vi "Rotation3D_Create_RotMatrix.vi"(11 "RotationMatrix":T1) -> (0 "Error":bool, 3 "Rotation3d":T2={"Q_quaternion"={"R"=1.0, "V"=[0.0, 0.0, 0.0]}})   [LabVIEW 2019, in "Trajectory_Library.lvlib"]
doc: "Constructs a Rotation3d from a rotation matrix.\n\nInputs::\n -- rotationMatrix -- The rotation matrix\n\nReturns:\n -- Rotation3d -- The created Rotation3d data cluster\n -- Error -- TRUE indicates an error occured."
uses:
  Trajectory_Library.lvlib
  TypeDef/ROTATION3D.ctl
  TypeDef/QUATERNION.ctl
  <vilib>/Analysis/Matrix/Datatypes/RealMatrix.ctl
  <vilib>/Analysis/baseanly.llb/Real A x B.vi
  <vilib>/Analysis/baseanly.llb/Real Determinant.vi
  Quaternion_Normalize.vi
  Quaternion_New_Default.vi
  <vilib>/Analysis/7linalg.llb/Create Special Matrix.vi
  <vilib>/Analysis/7linalg.llb/Create Special Real Matrix.vi
  <vilib>/Analysis/NI_AALBase.lvlib
  <vilib>/Analysis/Matrix/NI_Matrix.lvlib
  <vilib>/Analysis/Matrix/Numeric/Subtract/Subtract - RM,RM.vi
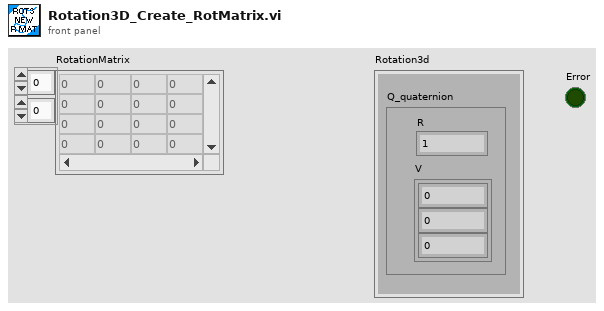
[diagram p1: front panel]
types:
  T1 = typedef "NI_Matrix.lvlib/RealMatrix.ctl" = dbl[][]
  T2 = typedef "Trajectory_Library.lvlib/ROTATION3D.ctl" = cluster{"Q_quaternion":T3}
  T3 = typedef "Trajectory_Library.lvlib/QUATERNION.ctl" = cluster{"R":dbl, "V":dbl[]}
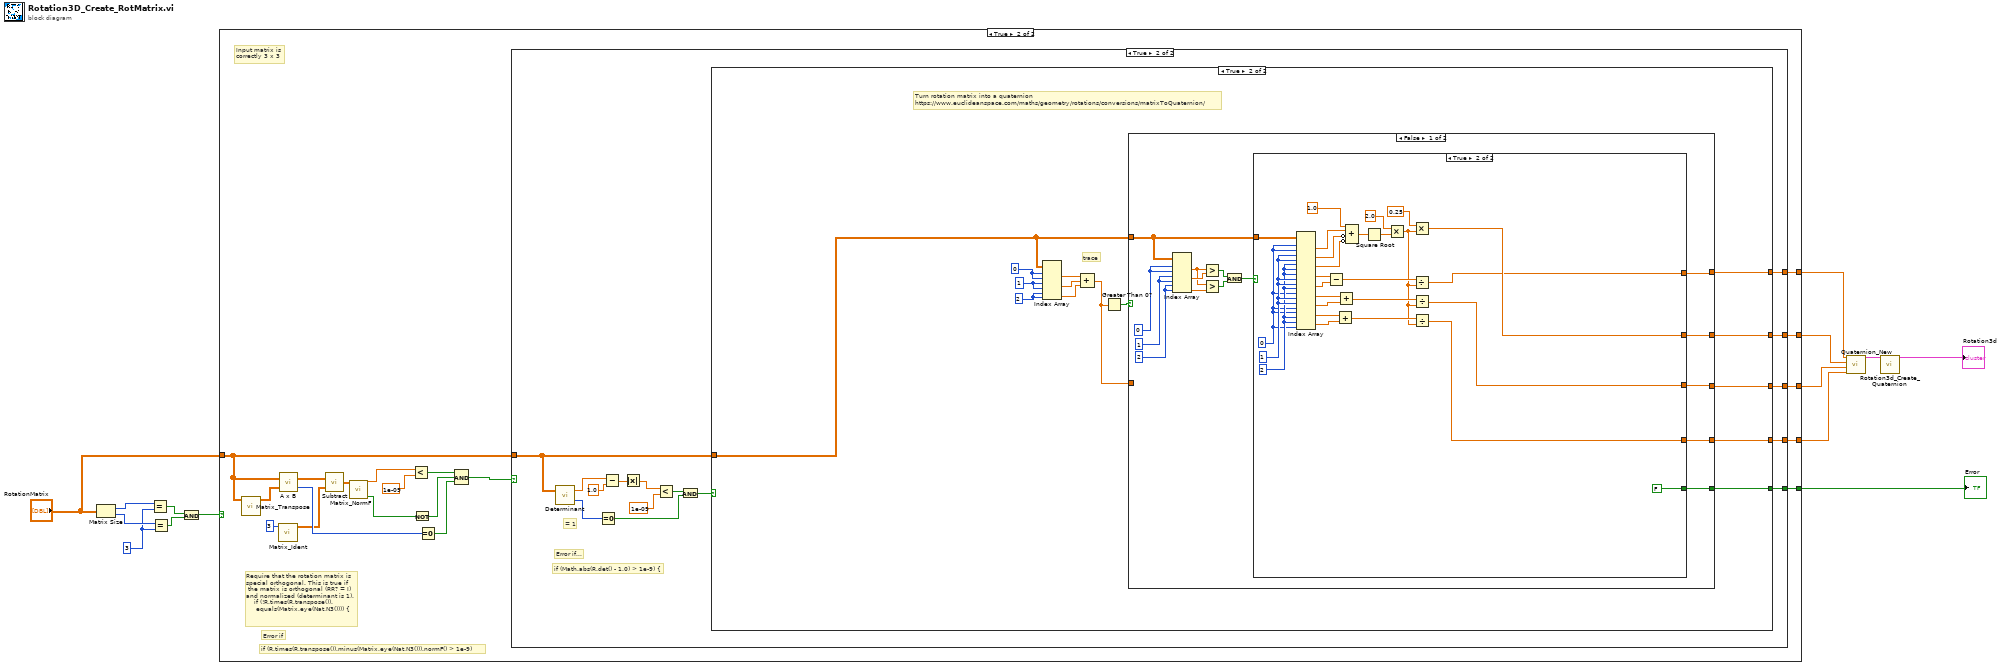
[diagram p0: block diagram]
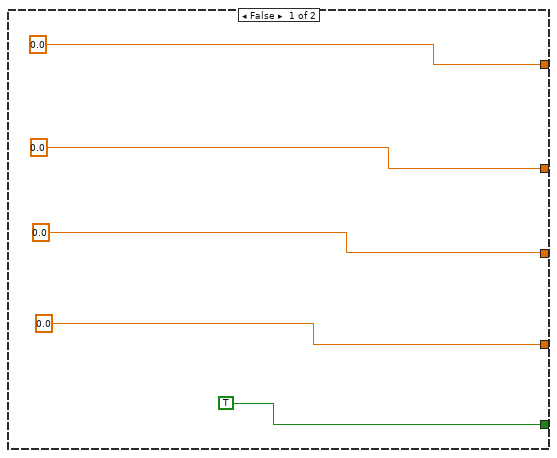
[diagram p2: hidden frame]
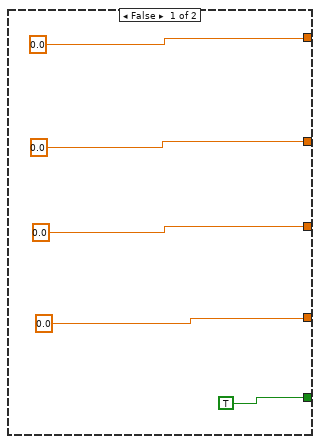
[diagram p3: hidden frame]
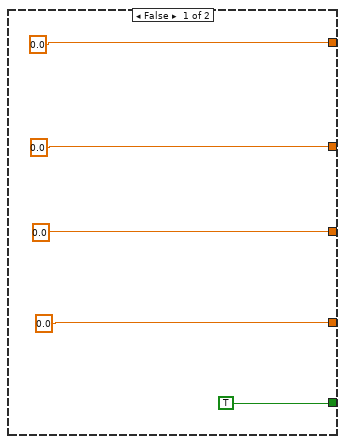
[diagram p4: hidden frame]
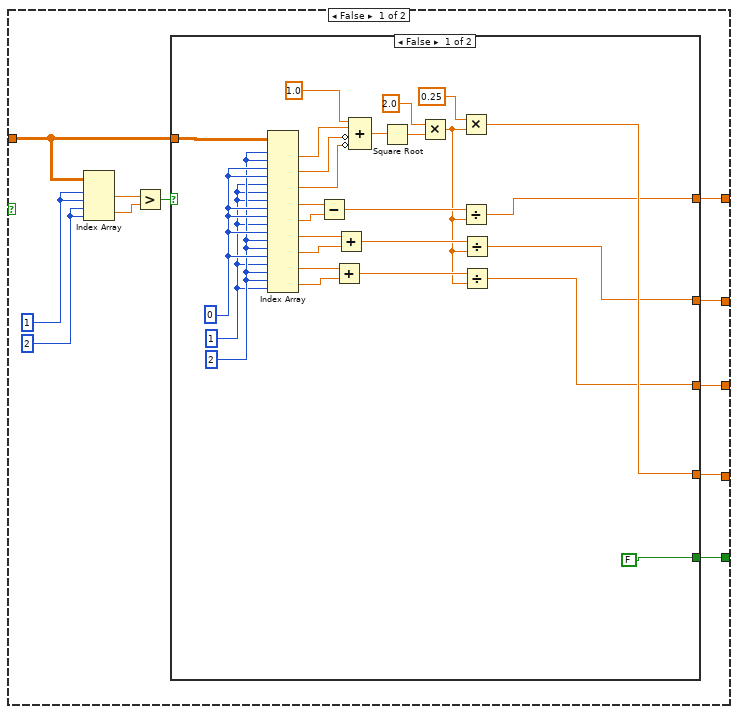
[diagram p5: hidden frame]
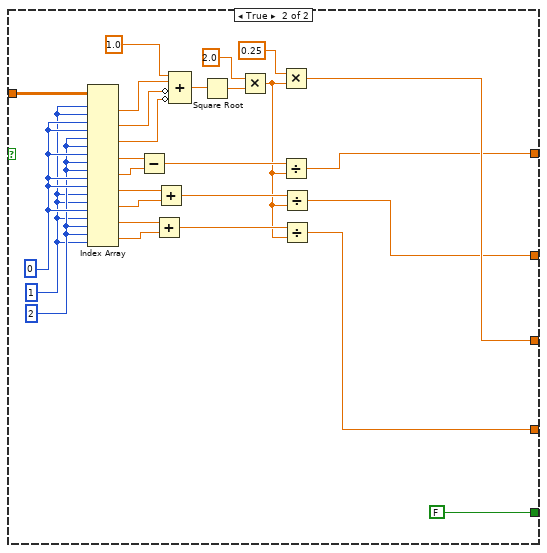
[diagram p6: hidden frame]
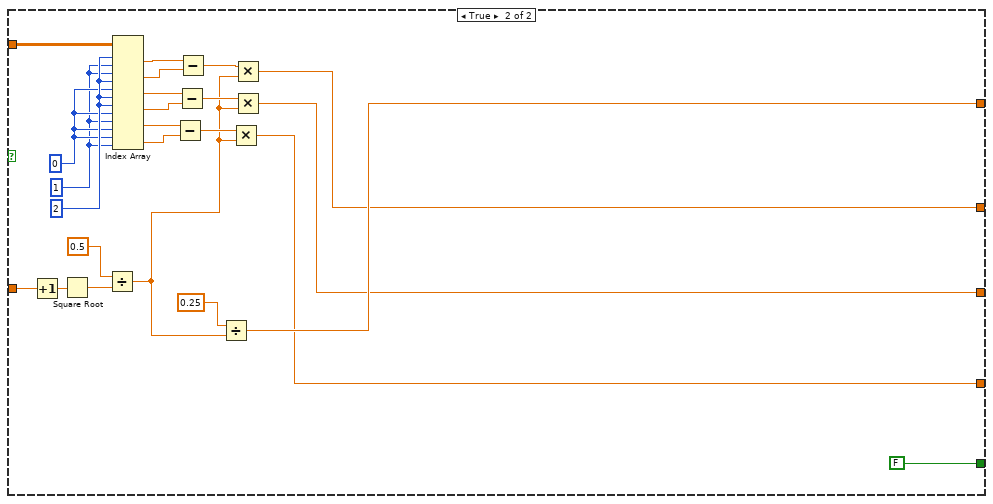
[diagram p7: hidden frame]
diagram:
  w7 = 3 ("y")
  n1 = Matrix Size(0:"RotationMatrix") -> (1:w9:i32, 2:w8:i32)
  n2 = Equal?(x=w9, y=w7) -> (x = y?=w5:bool)
  n3 = Equal?(x=w8, y=w7) -> (x = y?=w6:bool)
  n4 = And(x=w5, y=w6) -> (x .and. y?=w1:bool)
  n5 = case shown="True" w1 {
    tunnel: [0.0 w38] -> w13
    tunnel: [0.0 w37] -> w12
    tunnel: [0.0 w36] -> w11
    tunnel: [0.0 w35] -> w10
    tunnel: [TRUE w34] -> w4
    tunnel: "RotationMatrix" -> [_ w28]
    frame False {
    }
    frame True {
      # "if (R.times(R.transpose()).minus(Matrix.eye(Nat.N3())).normF() > 1e-9)"
      # "Error if"
      # "Require that the rotation matrix is \nspecial orthogonal. This is true if\n the matrix is orthogonal (RR? = I) \nand normalized (determinant is 1).\n    if (!R.times(R.transpose()).\n     equals(Matrix.eye(Nat.N3()))) {"
      # "Input matrix is \ncorrectly 3 x 3"
      n6 = call "Matrix_Transpose.vi"("input matrix"=w28) -> ("output matrix"=w33:T1)  [unwired: 10 in]
      n7 = call "Matrix_Ident.vi"("Size"=3) -> ("output matrix"=w26:T1)  [unwired: 9 in, 1 out]
      n8 = call-poly <vilib>:"A x B.vi"("B"=w33, "A"=w28) -> ("error"=w31:i32, "A x B"=w27:T1)
      n9 = call-poly <vilib>:"Subtract.vi"("Real Matrix B"=w26, "Real Matrix A"=w27) -> ("A - B"=w25:T1)
      n10 = call "Matrix_NormF.vi"("input matrix"=w25) -> ("Error"=w24:bool, "normF"=w21:dbl)  [unwired: 9 in]
      n11 = Less?(x=w21, y=1e-09) -> (x < y?=w22:bool)
      n12 = Not(x=w24) -> (.not. x?=w23:bool)
      n13 = Equal To 0?(x=w31) -> (x = 0?=w30:bool)
      n14 = Compound Arithmetic op=AND(w22, w23, w30) -> (w29:bool)
      n15 = case shown="True" w29 {
        tunnel: [0.0 w58] -> w38
        tunnel: [0.0 w57] -> w37
        tunnel: [0.0 w56] -> w36
        tunnel: [0.0 w55] -> w35
        tunnel: [TRUE w54] -> w34
        tunnel: w28 -> [_ w50]
        frame False {
        }
        frame True {
          # "Error if..."
          # "if (Math.abs(R.det() - 1.0) > 1e-9) {"
          # "= 1"
          n16 = call-poly <vilib>:"Determinant.vi"("Input Matrix"=w50) -> ("error"=w53:i32, "determinant"=w49:dbl)  [unwired: 1 in]
          n17 = Equal To 0?(x=w53) -> (x = 0?=w52:bool)
          n18 = Subtract(x=w49, y=1.0 ("x")) -> (x-y=w47:dbl)
          n19 = Absolute Value(x=w47) -> (abs(x)=w45:dbl)
          n20 = Less?(x=w45, y=1e-09) -> (x < y?=w46:bool)
          n21 = And(x=w46, y=w52) -> (x .and. y?=w51:bool)
          n22 = case shown="True" w51 {
            tunnel: [0.0 w77] -> w58
            tunnel: [0.0 w76] -> w57
            tunnel: [0.0 w75] -> w56
            tunnel: [0.0 w74] -> w55
            tunnel: [TRUE w73] -> w54
            tunnel: w50 -> [_ w72]
            frame False {
            }
            frame True {
              w69 = 2 ("index (row)")
              w70 = 1 ("index (row)")
              w71 = 0 ("index (row)")
              # "Turn rotation matrix into a quaternion\nhttps://www.euclideanspace.com/maths/geometry/rotations/conversions/matrixToQuaternion/"
              # "trace"
              n23 = Index Array(array=w72, index (row) #1=w71, index (col) #1=w71, index (row) #2=w70, index (col) #2=w70, index (row) #3=w69, index (col) #3=w69) -> (element #1=w68:dbl, element #2=w67:dbl, element #3=w66:dbl)
              n24 = Compound Arithmetic op=ADD(w68, w67, w66) -> (w64:dbl)
              n25 = Greater Than 0?(x=w64) -> (x > 0?=w65:bool)
              n26 = case shown="False" w65 {
                tunnel: w64 -> [_ w208]
                tunnel: w72 -> [w92 w204]
                tunnel: [w81 w202] -> w77
                tunnel: [w82 w188] -> w76
                tunnel: [w80 w187] -> w75
                tunnel: [w79 w186] -> w74
                tunnel: [w78 FALSE] -> w73
                frame False {
                  w88 = 2 ("index (row)")
                  w90 = 1 ("index (row)")
                  w91 = 0 ("index (row)")
                  n27 = Index Array(array=w92, index (row) #1=w91, index (col) #1=w91, index (row) #2=w90, index (col) #2=w90, index (row) #3=w88, index (col) #3=w88) -> (element #1=w87:dbl, element #2=w89:dbl, element #3=w86:dbl)
                  n28 = Greater?(x=w87, y=w89) -> (0:w84:bool)
                  n29 = Greater?(x=w87, y=w86) -> (0:w85:bool)
                  n30 = And(x=w84, y=w85) -> (x .and. y?=w83:bool)
                  n31 = case shown="True" w83 {
                    tunnel: w92 -> [w98 w184]
                    tunnel: [w95 w175] -> w82
                    tunnel: [w96 w171] -> w81
                    tunnel: [w97 w160] -> w80
                    tunnel: [w94 w159] -> w79
                    tunnel: [w93 FALSE] -> w78
                    frame False {
                      w100 = 2 ("index (row)")
                      w101 = 1 ("index (row)")
                      n32 = Index Array(array=w98, index (row) #1=w101, index (col) #1=w101, index (row) #2=w100, index (col) #2=w100) -> (element #1=w102:dbl, element #2=w103:dbl)
                      n33 = Greater?(x=w102, y=w103) -> (0:w99:bool)
                      n34 = case shown="False" w99 {
                        tunnel: w98 -> [w112 w139]
                        tunnel: [w105 w138] -> w97
                        tunnel: [w107 w134] -> w96
                        tunnel: [w106 w133] -> w95
                        tunnel: [w111 w132] -> w94
                        tunnel: [FALSE FALSE] -> w93
                        frame False {
                          w109 = 2 ("index (row)")
                          w108 = 1 ("index (row)")
                          w110 = 0 ("index (row)")
                          n35 = Index Array(array=w112, index (row) #1=w109, index (col) #1=w109, index (row) #2=w110, index (col) #2=w110, index (row) #3=w108, index (col) #3=w108, index (row) #4=w108, index (col) #4=w110, index (row) #5=w110, index (col) #5=w108, index (row) #6=w110, index (col) #6=w109, index (row) #7=w109, index (col) #7=w110, index (row) #8=w108, index (col) #8=w109, index (row) #9=w109, index (col) #9=w108) -> (element #1=w129:dbl, element #2=w128:dbl, element #3=w127:dbl, element #4=w122:dbl, element #5=w121:dbl, element #6=w119:dbl, element #7=w118:dbl, element #8=w117:dbl, element #9=w116:dbl)
                          n36 = Subtract ("Subtract.vi")(x=w122, y=w121) -> (x-y=w120:dbl)
                          n37 = Add ("Add.vi")(x=w117, y=w116) -> (x+y=w115:dbl)
                          n38 = Add ("Add.vi")(x=w119, y=w118) -> (x+y=w114:dbl)
                          n39 = Compound Arithmetic op=ADD(1.0, w129, invert w128, invert w127) -> (w126:dbl)
                          n40 = Square Root(x=w126) -> (sqrt(x)=w125:dbl)
                          n41 = Multiply(x=2.0, y=w125) -> (x*y=w113:dbl)
                          n42 = Multiply(x=0.25, y=w113) -> (x*y=w111:dbl)
                          n43 = Divide(x=w120, y=w113) -> (x/y=w107:dbl)
                          n44 = Divide(x=w114, y=w113) -> (x/y=w106:dbl)
                          n45 = Divide(x=w115, y=w113) -> (x/y=w105:dbl)
                        }
                        frame True {
                          w136 = 2 ("index (row)")
                          w135 = 1 ("index (row)")
                          w137 = 0 ("index (row)")
                          n46 = Index Array(array=w139, index (row) #1=w135, index (col) #1=w135, index (row) #2=w137, index (col) #2=w137, index (row) #3=w136, index (col) #3=w136, index (row) #4=w137, index (col) #4=w136, index (row) #5=w136, index (col) #5=w137, index (row) #6=w137, index (col) #6=w135, index (row) #7=w135, index (col) #7=w137, index (row) #8=w135, index (col) #8=w136, index (row) #9=w136, index (col) #9=w135) -> (element #1=w156:dbl, element #2=w155:dbl, element #3=w154:dbl, element #4=w149:dbl, element #5=w148:dbl, element #6=w146:dbl, element #7=w145:dbl, element #8=w144:dbl, element #9=w143:dbl)
                          n47 = Subtract ("Subtract.vi")(x=w149, y=w148) -> (x-y=w147:dbl)
                          n48 = Add ("Add.vi")(x=w144, y=w143) -> (x+y=w142:dbl)
                          n49 = Add ("Add.vi")(x=w146, y=w145) -> (x+y=w141:dbl)
                          n50 = Compound Arithmetic op=ADD(1.0, w156, invert w155, invert w154) -> (w153:dbl)
                          n51 = Square Root(x=w153) -> (sqrt(x)=w152:dbl)
                          n52 = Multiply(x=2.0, y=w152) -> (x*y=w140:dbl)
                          n53 = Multiply(x=0.25, y=w140) -> (x*y=w138:dbl)
                          n54 = Divide(x=w147, y=w140) -> (x/y=w134:dbl)
                          n55 = Divide(x=w141, y=w140) -> (x/y=w133:dbl)
                          n56 = Divide(x=w142, y=w140) -> (x/y=w132:dbl)
                        }
                      }
                    }
                    frame True {
                      w169 = 2 ("index (row)")
                      w170 = 1 ("index (row)")
                      w168 = 0 ("index (row)")
                      n57 = Index Array(array=w184, index (row) #1=w168, index (col) #1=w168, index (row) #2=w170, index (col) #2=w170, index (row) #3=w169, index (col) #3=w169, index (row) #4=w169, index (col) #4=w170, index (row) #5=w170, index (col) #5=w169, index (row) #6=w168, index (col) #6=w170, index (row) #7=w170, index (col) #7=w168, index (row) #8=w168, index (col) #8=w169, index (row) #9=w169, index (col) #9=w168) -> (element #1=w182:dbl, element #2=w181:dbl, element #3=w180:dbl, element #4=w174:dbl, element #5=w173:dbl, element #6=w167:dbl, element #7=w166:dbl, element #8=w165:dbl, element #9=w164:dbl)
                      n58 = Subtract(x=w174, y=w173) -> (x-y=w172:dbl)
                      n59 = Add(x=w165, y=w164) -> (x+y=w163:dbl)
                      n60 = Add(x=w167, y=w166) -> (x+y=w162:dbl)
                      n61 = Compound Arithmetic op=ADD(1.0, w182, invert w181, invert w180) -> (w179:dbl)
                      n62 = Square Root(x=w179) -> (sqrt(x)=w178:dbl)
                      n63 = Multiply(x=2.0, y=w178) -> (x*y=w161:dbl)
                      n64 = Multiply(x=0.25, y=w161) -> (x*y=w175:dbl)
                      n65 = Divide(x=w172, y=w161) -> (x/y=w171:dbl)
                      n66 = Divide(x=w162, y=w161) -> (x/y=w160:dbl)
                      n67 = Divide(x=w163, y=w161) -> (x/y=w159:dbl)
                    }
                  }
                }
                frame True {
                  w199 = 2 ("index (row)")
                  w197 = 1 ("index (row)")
                  w198 = 0 ("index (row)")
                  n68 = Increment(x=w208) -> (x+1=w207:dbl)
                  n69 = Square Root(x=w207) -> (sqrt(x)=w206:dbl)
                  n70 = Divide(x=0.5, y=w206) -> (x/y=w189:dbl)
                  n71 = Index Array(array=w204, index (row) #1=w199, index (col) #1=w197, index (row) #2=w197, index (col) #2=w199, index (row) #3=w198, index (col) #3=w199, index (row) #4=w199, index (col) #4=w198, index (row) #5=w197, index (col) #5=w198, index (row) #6=w198, index (col) #6=w197) -> (element #1=w201:dbl, element #2=w200:dbl, element #3=w196:dbl, element #4=w195:dbl, element #5=w194:dbl, element #6=w193:dbl)
                  n72 = Subtract(x=w194, y=w193) -> (x-y=w190:dbl)
                  n73 = Subtract(x=w196, y=w195) -> (x-y=w191:dbl)
                  n74 = Subtract(x=w201, y=w200) -> (x-y=w192:dbl)
                  n75 = Divide(x=0.25, y=w189) -> (x/y=w202:dbl)
                  n76 = Multiply(x=w190, y=w189) -> (x*y=w186:dbl)
                  n77 = Multiply(x=w192, y=w189) -> (x*y=w188:dbl)
                  n78 = Multiply(x=w191, y=w189) -> (x*y=w187:dbl)
                }
              }
            }
          }
        }
      }
    }
  }
  "Error" <- w4
  n79 = call "Quaternion_New.vi"("Z"=w10, "Y"=w11, "X"=w12, "W"=w13) -> ("out Quaternion"=w14:T3)  [unwired: 7 in]
  n80 = call "Rotation3d_Create_Quaternion.vi"("Quaternion"=w14) -> ("Rotation3d"=→"Rotation3d":T2)  [unwired: 10 in]
